vi "GetStringGlobalVariables.vi"(8 "error in (no error)":errorcluster, 9 "varCount":i32, 10 "varNumber":i32, 11 "controller in":refnum<k24>) -> (0 "error out":errorcluster, 2 "string values out":string[](array[string]), 3 "controller out":refnum<k24>)   [LabVIEW 2010]
uses:
  c:/aerotech/controller/5.xx.xxx/A3200/pc/labview/2010/bin/Aerotech.A3200.dll
  bin/Aerotech.A3200.dll
  c:/aerotech/controller/5.xx.xxx/A3200/pc/labview/2010/bin/Aerotech.A3200.LabVIEW.dll
  bin/Aerotech.A3200.LabVIEW.dll
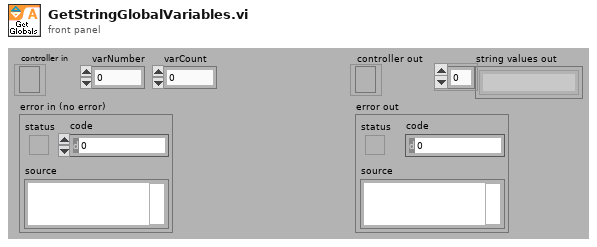
[diagram p1: front panel]
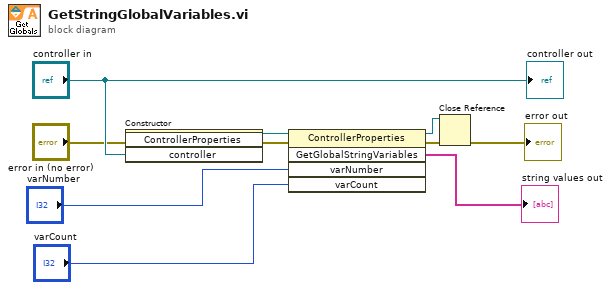
[diagram p0: block diagram]
diagram:
  n1 = constructor class="ControllerProperties"(error in="error in (no error)", "controller"="controller in") -> (reference out=w10:refnum<k24>, error out=w9:errorcluster)  [unwired: 2 in, 2 out]
  n2 = invoke class="ControllerProperties" method="GetGlobalStringVariables"(reference=w10, error in=w9, "varNumber"="varNumber", "varCount"="varCount") -> (reference out=w3:refnum<k24>, error out=w4:errorcluster, "GetGlobalStringVariables"=→"string values out":string[])  [unwired: 1 in, 2 out]
  n3 = Close Reference(reference=w3, error in (no error)=w4) -> (error out=→"error out":errorcluster)
  "controller out" <- "controller in"
